vi "openbci_sdcard_commands.vi"() -> ()   [LabVIEW 2013]
doc: "Send control commands to logging into the SD card"
uses:
  Control Def/openbci_device.ctl
  Control Def/channel_count.ctl
  Control Def/sd_log_times.ctl
panel:
  in  "SD Log times":T1=106 items=["5MIN"=65, "15MIN"=83, "30M"=70, "1HR"=71, "2HR"=72, "4HR"=74, "12HR"=75, "24HR"=76, "14SEC TEST"=97, "STOP"=106]
  in  "error in (no error)":errorcluster
  out "error out":errorcluster
  in  "OBCI dev in":T2={"COM port"="", "n_ch (8)"=enum."8 Channels", "delay_tx"=50}
  out "OBCI dev out":T2={"COM port"="", "n_ch (8)"=enum."8 Channels", "delay_tx"=50}
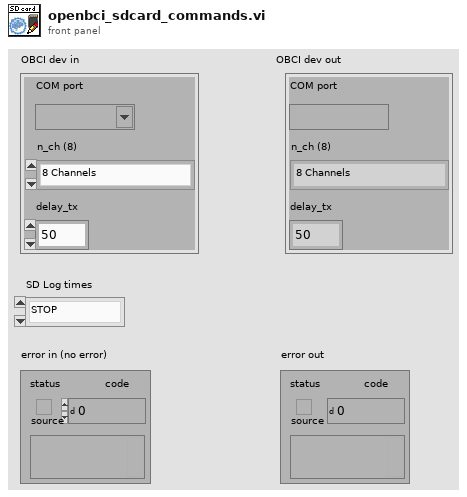
[diagram p1: front panel]
types:
  T1 = typedef "sd_log_times.ctl" = u16
  T2 = typedef "openbci_device.ctl" = cluster{"COM port":refnum<visa-resource-name>, "n_ch (8)":T3, "delay_tx":u32}
  T3 = typedef "channel_count.ctl" = enum16{"8 Channels", "16 Channels"}
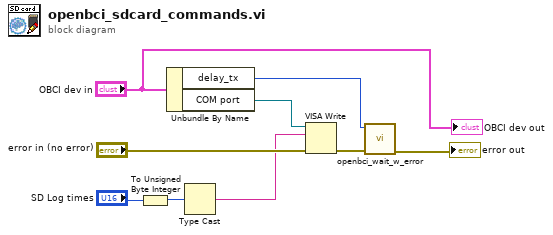
[diagram p0: block diagram]
diagram:
  n1 = To Unsigned Byte Integer(number="SD Log times") -> (unsigned 8bit integer=w9:u8)
  n2 = Unbundle By Name("OBCI dev in") -> ("delay_tx"=w2:u32, "COM port"=w8:refnum<visa-resource-name>)
  n3 = Type Cast(x=w9) -> (*(type *) &x=w5:string)  [unwired: 1 in]
  n4 = VISA Write(VISA resource name=w8, write buffer=w5, error in (no error)="error in (no error)") -> (error out=w4:errorcluster)  [unwired: 2 out]
  n5 = call "openbci_wait_w_error.vi"("error in (no error)"=w4, "milliseconds to wait"=w2) -> ("error out"=→"error out":errorcluster)  [unwired: 9 in]
  "OBCI dev out" <- "OBCI dev in"
